vi "Add Actor-Interface to Tree.vi"(0 "Message Maker in":refnum<class "Message Maker.lvclass">, 1 "Actor/Interface Refnum in":refnum<vi>, 5 "error in (no error)":errorcluster) -> (14 "Message Maker out":refnum<class "Message Maker.lvclass">, 15 "Actor/Interface Refnum out":refnum<vi>, 16 "Actor/Interface Tag":string, 17 "All Method Refnums":refnum<vi>[](array[refnum]), 19 "error out":errorcluster)   [LabVIEW 2023, in "Message Maker.lvclass"]
uses:
  Message Maker.lvclass
  Message Maker.lvclass/Message Maker.ctl
panel:
  out "TreeControl out":refnum<vi>
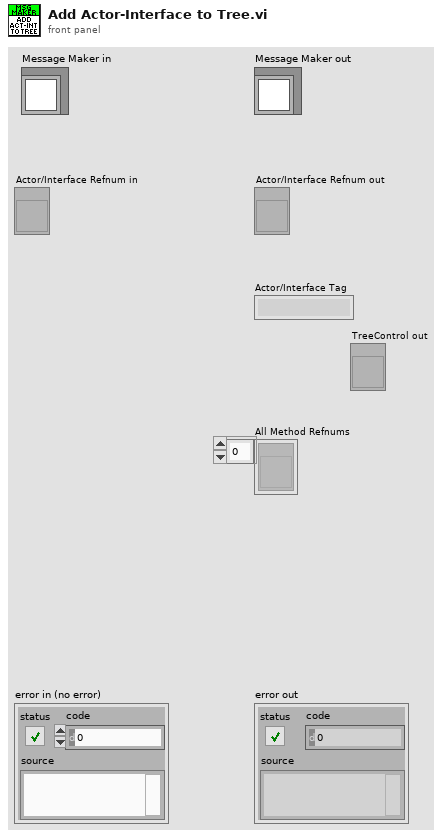
[diagram p1: front panel]
types:
  T1 = typedef "Message Maker.lvclass/Details Map.ctl" = map{string, string}
  T2 = typedef "Message Maker.lvclass/Message Recipient Type.ctl" = enum16{"Actor", "Interface", "Async Actor"}
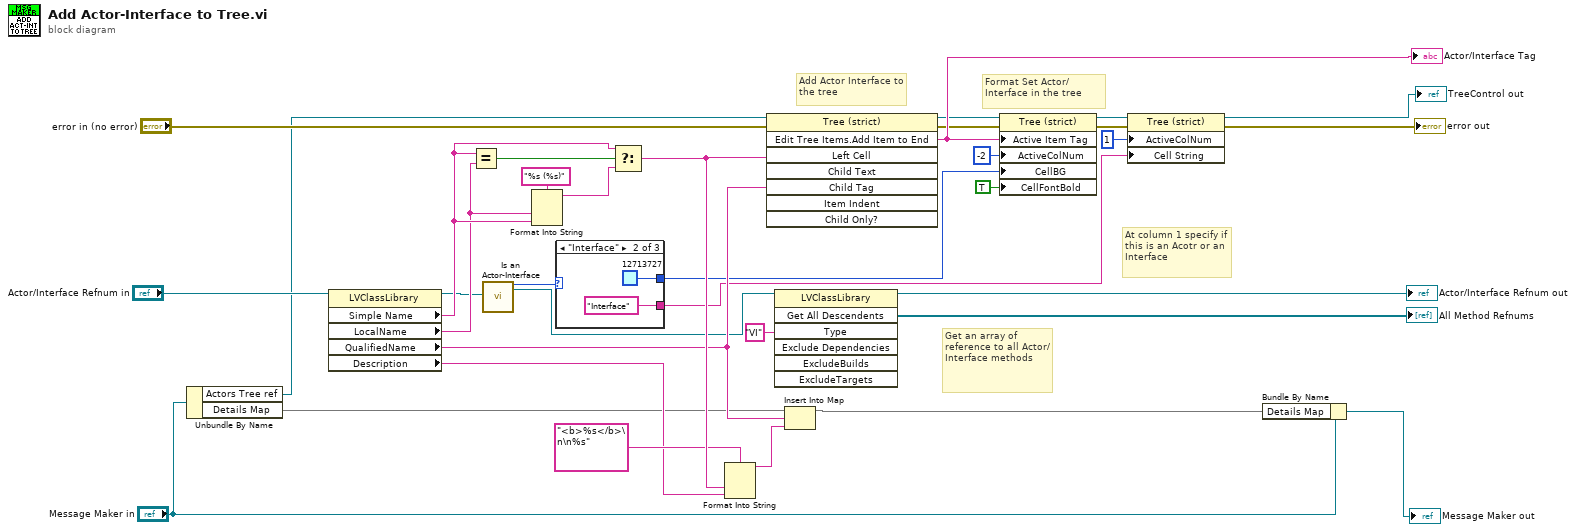
[diagram p0: block diagram]
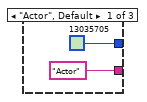
[diagram p2: hidden frame]
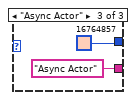
[diagram p3: hidden frame]
diagram:
  # "At column 1 specify if this is an Acotr or an Interface"
  # "Get an array of reference to all Actor/Interface methods"
  # "Format Set Actor/Interface in the tree"
  # "Add Actor Interface to the tree"
  n1 = Unbundle By Name("Message Maker in") -> ("Actors Tree ref"=w10:refnum<vi>, "Details Map"=w9:T1)
  n2 = property class="LVClassLibrary"(reference="Actor/Interface Refnum in") -> (reference out=w6:refnum<vi>, "Simple Name"=w23:string, "LocalName"=w22:string, "QualifiedName"=w25:string, "Description"=w16:string)  [unwired: 1 in, 1 out]
  n3 = Equal?(x=w23, y=w22) -> (x = y?=w19:bool)
  n4 = call "Is an Actor-Interface.vi"("Class in"=w6) -> ("Message Recipient Type"=w4:T2, "Class out"=w5:refnum<vi>)  [unwired: 14 in, 3 out]
  n5 = Format Into String(format string="%s (%s)", w22, w23) -> (resulting string=w21:string)  [unwired: 2 in, 1 out]
  n6 = case shown="\"Interface\"" w4 {
    tunnel: ["Actor" ("format string") "Interface" ("format string") "Async Actor" ("format string")] -> w2
    tunnel: [u32 13035705 u32 12713727 u32 16764857] -> w3
    frame "Actor", Default {
    }
    frame "Interface" {
    }
    frame "Async Actor" {
    }
  }
  n7 = Select(t=w23, s=w19, f=w21) -> (s? t:f=w32:string)
  n8 = Format Into String(format string="<b>%s</b>\n\n%s", w32, w16) -> (resulting string=w15:string)  [unwired: 2 in, 1 out]
  n9 = invoke class="Tree (strict)" method="Edit Tree Items.Add Item to End"(reference=w10, error in="error in (no error)", "Left Cell"=w32, "Child Tag"=w25) -> (reference out=w24:refnum<vi>, error out=w26:errorcluster, "Edit Tree Items:Add Item to End"=w33:string)  [unwired: 4 in, 5 out]
  "Actor/Interface Tag" <- w33
  n10 = invoke class="LVClassLibrary" method="Get All Descendents"(reference=w5, "Type"="VI") -> (reference out=→"Actor/Interface Refnum out":refnum<vi>, "All Descendents"=→"All Method Refnums":refnum<vi>[])  [unwired: 5 in, 5 out]
  n11 = Insert Into Map(map in=w9, key=w25, value=w15) -> (map out=w1:T1)  [unwired: 2 out]
  n12 = property on="Property Node" class="Tree (strict)"(reference=w24, error in=w26, "Active Item Tag"=w33, "ActiveColNum"=-2 ("Active Cell:Active Column Number"), "CellBG"=w3, "CellFontBold"=TRUE ("Active Cell:Cell Font:Bold")) -> (reference out=w35:refnum<vi>, error out=w29:errorcluster)
  n13 = property on="Property Node" class="Tree (strict)"(reference=w35, error in=w29, "ActiveColNum"=1 ("Active Cell:Active Column Number"), "Cell String"=w2) -> (reference out=→"TreeControl out":refnum<vi>, error out=→"error out":errorcluster)
  n14 = Bundle By Name(cluster="Message Maker in", "Details Map"=w1) -> (→"Message Maker out":refnum<class "Message Maker.lvclass">)
